vi "PH_Timing.PC Slow Trigger.vi"(0 "i ref in":refnum<vi>, 2 "Slow Trigger Settings":T1, 5 "error IO":errorcluster) -> (14 "i ref out":refnum<vi>, 19 "error out":errorcluster)   [LabVIEW 2014, in "PH_Timing.lvlib"]
doc: "This is a certain process case of Timing."
uses:
  PH_Timing.lvlib
  PH_Timing.Slow Trigger Settings.ctl
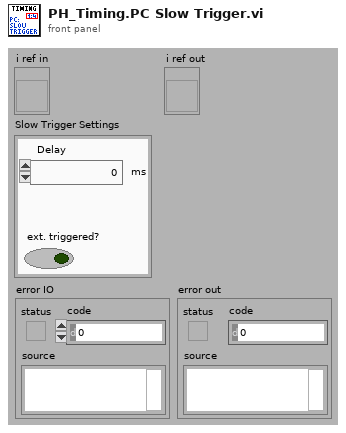
[diagram p1: front panel]
types:
  T1 = typedef "PH_Timing.lvlib/PH_Timing.Slow Trigger Settings.ctl" = cluster{"Delay":dbl, "externally triggered?":bool}
  T2 = typedef "PH_Timing.lvlib/PH_Timing.i attribute.ctl" = cluster{"Sequencer":cluster{"linked?":bool, "Proc State":string, "Ref State":refnum<vi>}, "Gate Generator":cluster{"GD":cluster{"Device Status":T3, "linked?":bool}, "Settings":T4, "GUI Ref":refnum<vi>}, "Interlock Bypass":cluster{"Instancename":string, "Switch linked?":bool, "Device Status":T3, "Ref Status":refnum<vi>}, "Roughtuner":cluster{"Settings":T5, "GUI Ref":refnum<vi>, "GD":cluster{"Device Status":T3, "linked?":bool}}, "0,5Hz Gater":cluster{"Settings":T6, "GUI Ref":refnum<vi>, "GD":cluster{"Device Status":T3, "linked?":bool}}, "Slow Trigger":cluster{"Settings":T1, "GUI Ref":refnum<vi>, "Service ID Delay":i32, "Service ID Ext Trig":i32, "Wanted Settings":T1}, "Timing Mode":cluster{"Mode":T7, "GUI Ref":refnum<vi>, "Service ID T2":i32, "Service ID Mode":i32, "Wanted Mode":T7}, "ns Generator":cluster{"Settings":T8, "ns Generator Settings":refnum<vi>, "GD":cluster{"Device Status":T3, "linked?":bool}}, "Phase FEs":cluster{"Settings":T11, "GUI Ref":refnum<vi>, "Service ID Phase":i32, "Wanted Settings":T11}, "GD GUI Refs":refnum<vi>[], "Heads":T12[], "GUI Ref Delete":refnum<vi>}
  T3 = typedef "PH_StatusHandler.lvlib/PH_StatusHandler.Status.ctl" = i16
  T4 = typedef "PH_Timing.lvlib/PH_Timing.GateGen.ctl" = cluster{"Instance":string, "Channel Gate":i32, "Channel T2":i32, "Width Gate":dbl, "Width T2":dbl, "Delay Gate":dbl, "Delay T2":dbl, "Gate activ":bool, "T2 activ":bool, "System Mode":enum16{"Normal", "Single", "Burst", "Duty Cycle"}}
  T5 = typedef "PH_Timing.lvlib/PH_Timing.Roughtuner.ctl" = cluster{"Instance":string, "Phase PHELIX / UNILAC":cluster{"Channel":u16, "relative to":u16, "Delay [ms]":dbl}, "Pulse Length":cluster{"Channel":u16, "relative to":u16, "Delay [ms]":dbl}, "Trigger":cluster{"externally?":bool, "Rate [Hz]":dbl}}
  T6 = typedef "PH_Timing.lvlib/PH_Timing.0.5HzGater.ctl" = cluster{"Instance":string, "Channel ns FE Delay":i32, "Channel 0.5Hz":i32, "Width ns FE Delay":dbl, "Width 0.5Hz":dbl, "Delay ns FE Delay":dbl, "Delay 0.5Hz":dbl, "ns FE Delay active":bool, "0.5Hz activ":bool, "ns FE Delay inverted":bool, "0.5Hz inverted":bool}
  T7 = typedef "PH_Timing.lvlib/PH_Timing.Timing Mode.ctl" = cluster{"T2":i16, "Modeselector":enum32{"10 Hz", "0.5 Hz", "Shot"}}
  T8 = typedef "PH_Timing.lvlib/PH_Timing.ns Generator.ctl" = cluster{"Instance":string, "Phase fs / ns FE":cluster{"Channel":T9, "Settings":T10}}
  T9 = typedef "Stanford Research DG645 - Driver.lvlib/Channel.ctl" = i32
  T10 = typedef "PH_SRDG645.lvlib/PH_SRDG645.Channel Settings.ctl" = cluster{"Delay [s]":dbl, "relative to":i32}
  T11 = typedef "PH_Timing.lvlib/PH_Timing.Phase FEs.ctl" = cluster{"Phase":dbl}
  T12 = typedef "PH_Timing.lvlib/PH_Timing.PU Data.ctl" = cluster{"linked?":bool, "Data":T13, "GD":cluster{"Device Status":T3, "linked?":bool}, "GUI Ref":refnum<vi>, "PU":T14}
  T13 = typedef "PH_Timing.lvlib/PH_Timing.PU Info.ctl" = cluster{"Act CH?":bool, "GD":string, "CH":i32, "Delay":dbl, "active":bool, "in Use?":bool}
  T14 = typedef "PH_PP_Common.lvlib/PH_PP_Common.PUs.ctl" = enum16{"no Info", "PA-19mm-1", "PA-19mm-2", "PA-45mm-PILC", "PA-45mm-MAIN", "MA-PU-1", "MA-PU-2", "MA-PU-3", "MA-PU-4", "MA-PU-5", "MA-PU-6", "MA-FR", "MA-PILC", "PA-45mm-DP"}
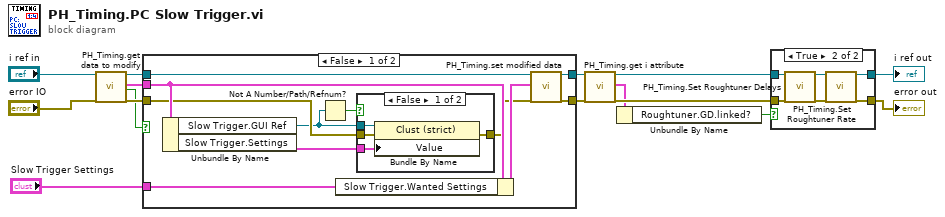
[diagram p0: block diagram]
diagram:
  n1 = call "PH_Timing.get data to modify.vi"("i ref in"="i ref in", "error in (no error)"="error IO") -> ("i ref out"=w13:refnum<vi>, "i attribute"=w11:T2, "timed out"=w10:bool, "error out"=w12:errorcluster)  [unwired: 14 in]
  n2 = case shown="False" w10 {
    tunnel: w13 -> [w26 w33]
    tunnel: [w25 w33] -> w6
    tunnel: w12 -> [w19 w32]
    tunnel: [w24 w32] -> w5
    tunnel: w11 -> [w21 _]
    tunnel: "Slow Trigger Settings" -> [w22 _]
    frame False {
      n3 = Unbundle By Name(w21) -> ("Slow Trigger.GUI Ref"=w16:refnum<vi>, "Slow Trigger.Settings"=w20:T1)
      n4 = Not A Number/Path/Refnum?(number/path/refnum=w16) -> (NaN/Path/Refnum?=w17:bool)
      n5 = Bundle By Name(cluster=w21, "Slow Trigger.Wanted Settings"=w22) -> (w23:T2)
      n6 = case shown="False" w17 {
        tunnel: w16 -> [w30 _]
        tunnel: w20 -> [w29 _]
        tunnel: w19 -> [w28 w31]
        tunnel: [w27 w31] -> w18
        frame False {
          n7 = property class="Clust (strict)"(reference=w30, error in=w28, "Value"=w29) -> (error out=w27:errorcluster)  [unwired: 1 out]
        }
        frame True {
        }
      }
      n8 = call "PH_Timing.set modified data.vi"("i ref in"=w26, "i attribute"=w23, "error in (no error)"=w18) -> ("i ref out"=w25:refnum<vi>, "error out"=w24:errorcluster)  [unwired: 15 in]
    }
    frame True {
    }
  }
  n9 = call "PH_Timing.get i attribute.vi"("i ref in"=w6, "error in (no error)"=w5) -> ("i ref out"=w8:refnum<vi>, "i attribute"=w7:T2, "error out"=w9:errorcluster)  [unwired: 15 in]
  n10 = Unbundle By Name(w7) -> ("Roughtuner.GD.linked?"=w1:bool)
  n11 = case shown="True" w1 {
    tunnel: w9 -> [w34 w40]
    tunnel: w8 -> [w35 w41]
    tunnel: [w34 w36] -> w3
    tunnel: [w35 w38] -> w4
    frame False {
    }
    frame True {
      n12 = call "PH_Timing.Set Roughtuner Delays.vi"("i ref in"=w41, "error in"=w40) -> ("i ref out"=w39:refnum<vi>, "error out"=w37:errorcluster)  [unwired: 16 in]
      n13 = call "PH_Timing.Set Roughtuner Rate.vi"("i ref in"=w39, "error in (no error)"=w37) -> ("i ref out"=w38:refnum<vi>, "error out"=w36:errorcluster)  [unwired: 16 in]
    }
  }
  "error out" <- w3
  "i ref out" <- w4
